vi "Parse.vi"(7 "channel blocks":T1[](array[typedef]) {"dst buffer offset" format="%d bytes"; "src buffer offset" format="%d bytes"}, 8 "error in (no error)":errorcluster, 10 "src Buffer":refnum<class "Buffer.lvclass">, 11 "Buffer Converter in":refnum<class "Buffer Converter.lvclass">) -> (0 "error out":errorcluster, 3 "Buffer Converter out":refnum<class "Buffer Converter.lvclass">)   [LabVIEW 2017, in "DSF Core.lvlib" / "Buffer Converter.lvclass"]
uses:
  Buffer Converter.lvclass
  Buffer/Buffer.lvclass
  DSF Configuration API/Public/Controls/DSF Engine Channel Configuration.ctl
  DSF Configuration API/Public/Controls/DSF Data Type.ctl
  DSF Core.lvlib
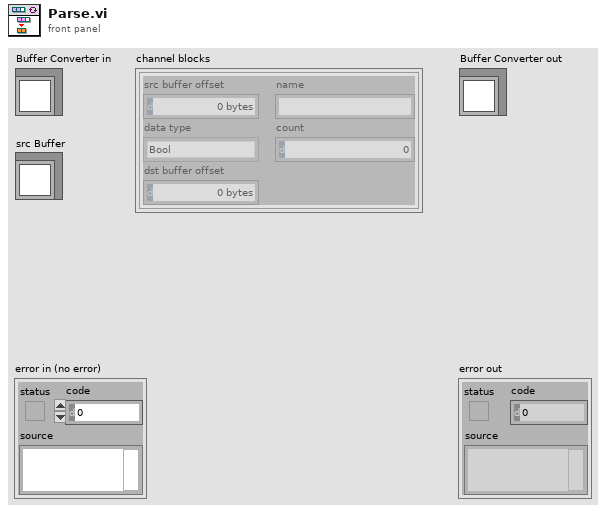
[diagram p1: front panel]
types:
  T1 = typedef "DSF Core.lvlib/DSF Engine Channel Configuration.ctl" = cluster{"src buffer offset":u64, "name":string, "data type":T2, "count":u64, "dst buffer offset":u64}
  T2 = typedef "DSF Core.lvlib/DSF Data Type.ctl" = enum8{"Bool", "SGL", "DBL", "I8", "I16", "I32", "I64", "U8", "U16", "U32", "U64"}
  T3 = typedef "DSF Core.lvlib/DSF Runtime Type Buffers.ctl" = cluster{"Bool":bool[], "SGL":sgl[], "DBL":dbl[], "I8":i8[], "I16":i16[], "I32":i32[], "I64":i64[], "U8":u8[], "U16":u16[], "U32":u32[], "U64":u64[]}
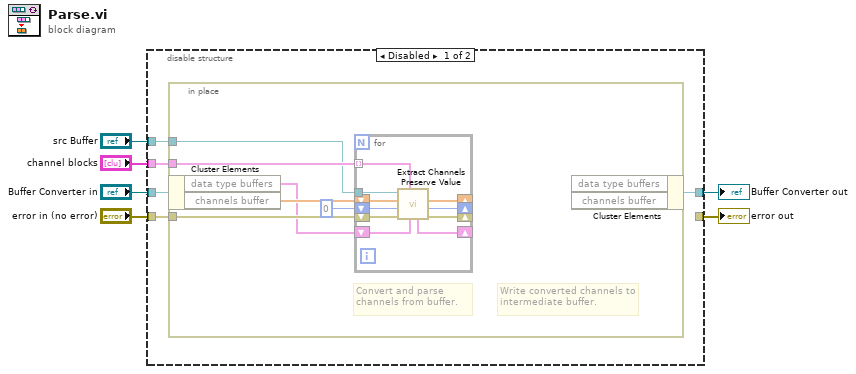
[diagram p0: block diagram]
diagram:
  n1 = disable-structure shown="Disabled" {
    disable-tunnel: "Buffer Converter in" -> [w11 w29]
    disable-tunnel: [w10 w29] -> w5
    disable-tunnel: "error in (no error)" -> [w9 w28]
    disable-tunnel: "src Buffer" -> [w8 _]
    disable-tunnel: "channel blocks" -> [w7 _]
    disable-tunnel: [_ w28] -> w1
    frame Disabled {
      n2 = in-place {
        in-place-border: w7 -> [w14]
        in-place-border: w9 -> [w15]
        in-place-border: w8 -> [w13]
        # "Write converted channels to intermediate buffer."
        # "Convert and parse channels from buffer."
        n3 = in-place-cluster #1(w11) -> ("data type buffers"=w12:T3, "channels buffer"=w16:dbl[])
        n4 = for {
          shift-right: [w26] -> _
          shift-left: w16 -> [w24]
          shift-right: [w27] -> _
          shift-left: w15 -> [w25]
          tunnel: w13 -> [w23]
          tunnel: w14 -> [w20] mode=indexing
          shift-right: [w22] -> _
          shift-left: w12 -> [w21]
          shift-right: [w19] -> _
          shift-left: u64 0 ("channels buffer index in") -> [w18]
          n5 = call "Extract Channels Preserve Value.vi"("data type buffers in"=w21, "channel block"=w20, "error in (no error)"=w25, "channels buffer index in"=w18, "channels buffer in"=w24, "Buffer in"=w23) -> ("error out"=w27:errorcluster, "channels buffer index out"=w19:u64, "channels buffer out"=w26:dbl[], "data type buffers out"=w22:T3)  [unwired: 1 in, 1 out]
        }
        n6 = in-place-cluster #1() -> (w10:refnum<class "Buffer Converter.lvclass">)  [unwired: 2 in]
      }
    }
    frame Enabled {
    }
  }
  "error out" <- w1
  "Buffer Converter out" <- w5
